vi "visitCircle.vi"(8 "error in (no error)":errorcluster, 10 "Circle":refnum<class "Circle.lvclass">, 11 "XMLExportVisitor in":refnum<class "XMLExportVisitor.lvclass">) -> (0 "error out":errorcluster, 2 "xml String":string, 3 "XMLExportVisitor out":refnum<class "XMLExportVisitor.lvclass">)   [LabVIEW 2018, in "XMLExportVisitor.lvclass"]
uses:
  XMLExportVisitor.lvclass
  Circle Class/Circle.lvclass
  Circle Class/Circle.lvclass/Circle.ctl
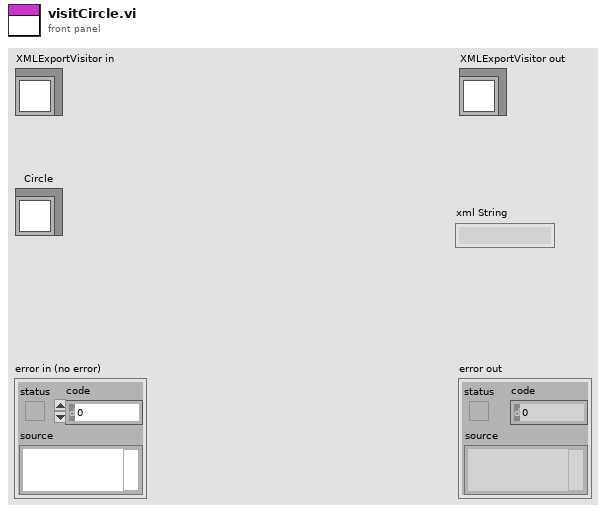
[diagram p1: front panel]
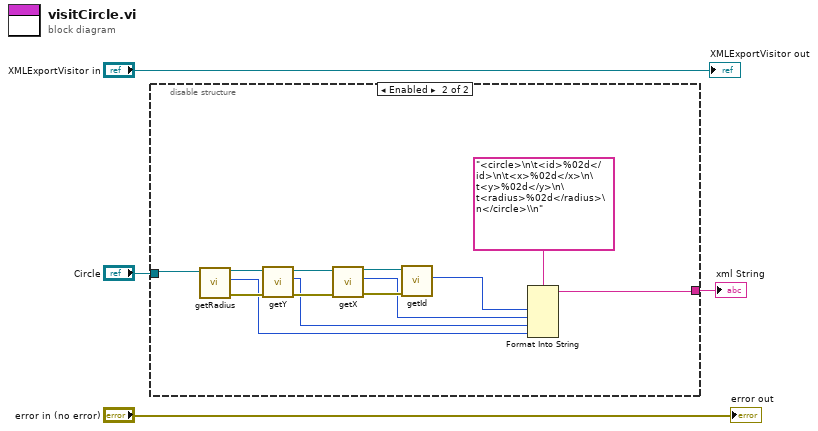
[diagram p0: block diagram]
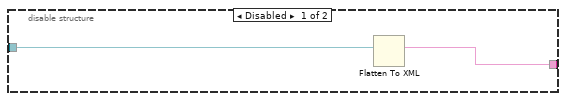
[diagram p2: hidden frame]
diagram:
  n1 = disable-structure shown="Enabled" {
    disable-tunnel: "Circle" -> [w6 w15]
    disable-tunnel: [w5 w7] -> w1
    frame Disabled {
      n2 = Flatten To XML(anything=w6) -> (xml string=w5:string)
    }
    frame Enabled {
      n3 = call "getRadius.vi"("Circle in"=w15) -> ("error out"=w18:errorcluster, "radius"=w8:i32, "Circle out"=w19:refnum<class "Circle.lvclass">)  [unwired: 8 in]
      n4 = call "getY.vi"("error in (no error)"=w18, "Circle in"=w19) -> ("error out"=w16:errorcluster, "y"=w9:i32, "Circle out"=w17:refnum<class "Circle.lvclass">)  [unwired: 7 in]
      n5 = call "getX.vi"("error in (no error)"=w16, "Circle in"=w17) -> ("error out"=w12:errorcluster, "x"=w10:i32, "Circle out"=w13:refnum<class "Circle.lvclass">)  [unwired: 7 in]
      n6 = call "getId.vi"("error in (no error)"=w12, "Circle in"=w13) -> ("id"=w11:i32)  [unwired: 7 in, 2 out]
      n7 = Format Into String(format string="<circle>\n\t<id>%02d</id>\n\t<x>%02d</x>\n\t<y>%02d</y>\n\t<radius>%02d</radius>\n</circle>\\n", w11, w10, w9, w8) -> (resulting string=w7:string)  [unwired: 2 in, 1 out]
    }
  }
  "xml String" <- w1
  "error out" <- "error in (no error)"
  "XMLExportVisitor out" <- "XMLExportVisitor in"
